vi "global_output.vi"() -> ()   [LabVIEW 2017]
panel:
  in  "Output Movement":T1(ring)
  in  "Output Speed":dbl
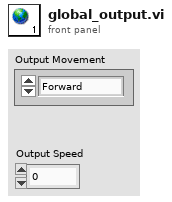
[diagram p1: front panel]
types:
  T1 = enum16{"Forward", "Backward", "Left", "Right", "Rotate Left", "Rotate Right"}
diagram:
